vi "Асинхронный ввод вывод for galvo.vi"() -> ()   [LabVIEW 2016]
panel:
  out "Канал АЦП 1":dbl(knob) scale=-2.0..2.0 scale format="%.1f"
  in  "milliseconds to wait":u32=100
  in  "ЦАП 2":dbl(slide)=-0.02227084646660238 scale=-2.0..2.0 scale format="%.1f"
  out "Module name":string
  in  "ЦАП":dbl(slide)=-0.11982121958747705 scale=-1.0..2.0 scale format="%.1f"
  in  "stop":bool
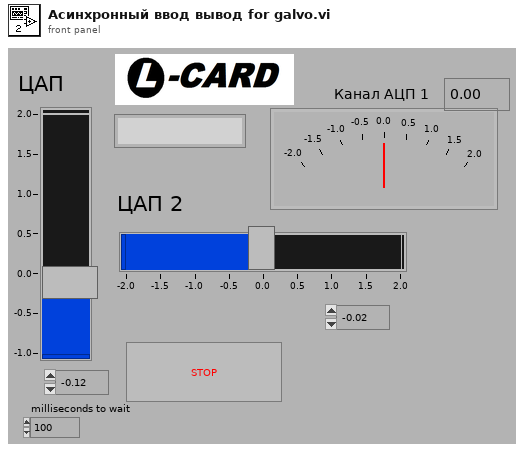
[diagram p1: front panel]
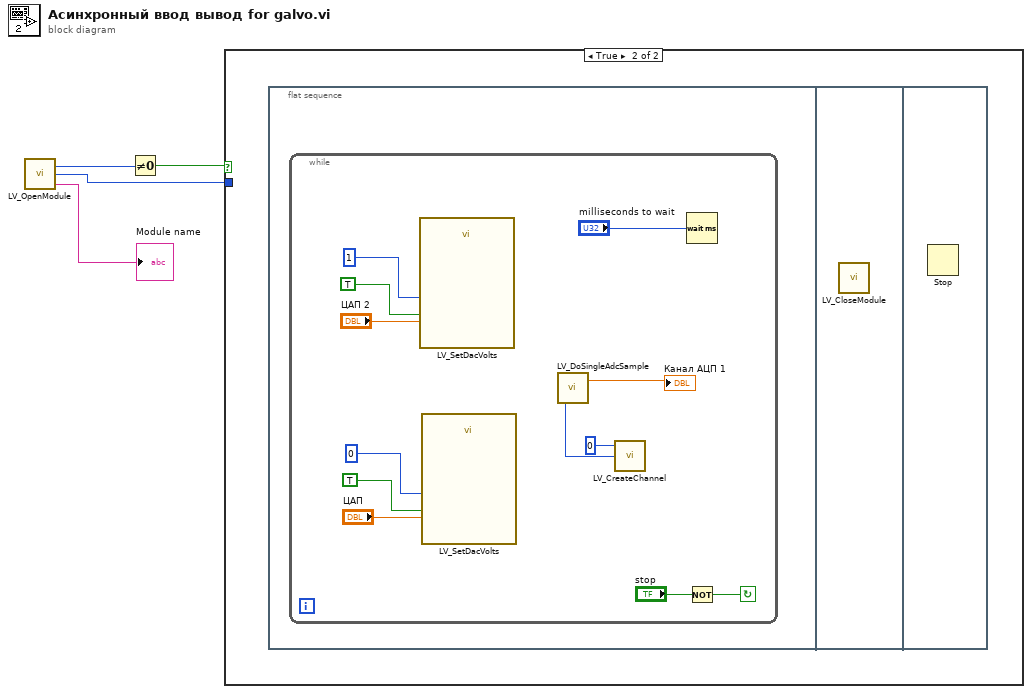
[diagram p0: block diagram]
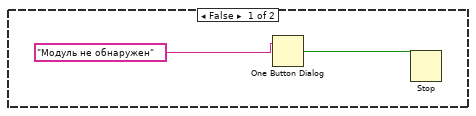
[diagram p2: hidden frame]
diagram:
  n1 = call "LV_OpenModule.vi"() -> ("Module Name"=→"Module name":string, "Module id"=w2:u8, "Error"=w3:u8)
  n2 = Not Equal To 0?(x=w3) -> (x != 0?=w4:bool)
  n3 = case shown="True" w4 {
    tunnel: w2 -> [_ _]
    frame False {
      n4 = One Button Dialog(message="Модуль не обнаружен") -> (true=w5:bool)  [unwired: 1 in]
      n5 = Stop(stop? (T)=w5) -> ()
    }
    frame True {
      n6 = flat-sequence {
        frame #0 {
          n7 = while {
            stop <- w17 continue-if-true
            n8 = stacked-sequence {
              frame #0 {
              }
              frame #1 {
              }
            }
            n9 = call <instrlib>:"LV_SetDacVolts.vi"("Voltage"="ЦАП 2", "Use calibr"=TRUE, "Channel Num"=1) -> ()
            n10 = call <instrlib>:"LV_SetDacVolts.vi"("Voltage"="ЦАП", "Use calibr"=TRUE, "Channel Num"=0) -> ()
            n11 = call <instrlib>:"LV_CreateChannel.vi"("Channel"=u16 0) -> ("Logical channel"=w8:u16)  [unwired: 2 in]
            n12 = call <instrlib>:"LV_DoSingleAdcSample.vi"("Logical ch Num"=w8) -> ("Result"=→"Канал АЦП 1":dbl)  [unwired: 1 in, 1 out]
            n13 = Wait (ms)(milliseconds to wait="milliseconds to wait") -> ()  [unwired: 1 out]
            n14 = Not(x="stop") -> (.not. x?=w17:bool)
          }
        }
        frame #1 {
          n15 = call "LV_CloseModule.vi"() -> ()  [unwired: 1 in]
        }
        frame #2 {
          n16 = Stop() -> ()  [unwired: 1 in]
        }
      }
    }
  }
